vi "NI VeriStand - Get System Node Children.vi"(8 "error in (no error)":errorcluster, 10 "Node":string, 11 "WorkspaceManager in":T3) -> (0 "error out":errorcluster {"code" format="%.0x"}, 2 "Nodes":T1[](array[typedef]), 3 "WorkspaceManager out":T3)   [LabVIEW 2020, in "NI_VS Workspace ExecutionAPI.lvlib"]
doc: "Returns information about the nodes directly under the specified system node."
uses:
  <vilib>/NI VeriStand/Execution/Workspace/NI_VS Workspace ExecutionAPI.lvlib
  <vilib>/NI VeriStand/Execution/Workspace/WorkspaceAPI.ctl
  NationalInstruments.VeriStand.ClientAPI
  <vilib>/NI VeriStand/Execution/Workspace/NodeInfo.ctl
  <vilib>/NI VeriStand/Execution/Workspace/Waveform Data Type.ctl
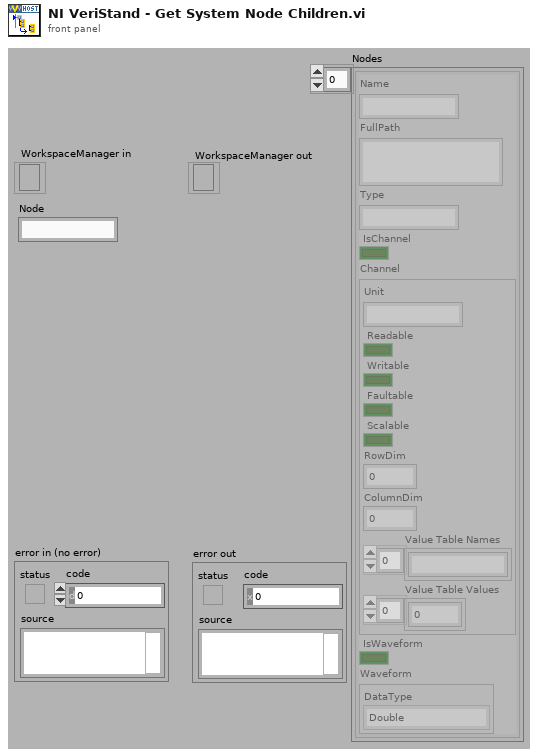
[diagram p1: front panel]
types:
  T1 = typedef "NI_VS Workspace ExecutionAPI.lvlib/NodeInfo.ctl" = cluster{"Name":string, "FullPath":string, "Type":string, "IsChannel":bool, "Channel":cluster{"Unit":string, "Readable":bool, "Writable":bool, "Faultable":bool, "Scalable":bool, "RowDim":u32, "ColumnDim":u32, "Value Table Names":string[], "Value Table Values":dbl[]}, "IsWaveform":bool, "Waveform":cluster{"DataType":T2}}
  T2 = typedef "NI_VS Workspace ExecutionAPI.lvlib/Waveform Data Type.ctl" = enum16{"Double", "ComplexDouble"}
  T3 = typedef "NI_VS Workspace ExecutionAPI.lvlib/WorkspaceAPI.ctl" = refnum<k24>
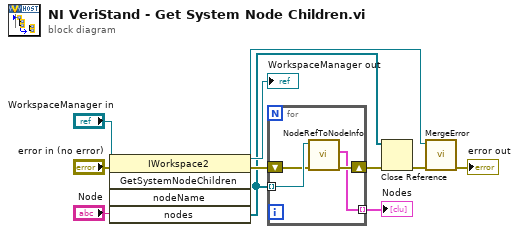
[diagram p0: block diagram]
diagram:
  n1 = invoke class="IWorkspace2" method="GetSystemNodeChildren"(reference="WorkspaceManager in", error in="error in (no error)", "nodeName"="Node") -> (reference out=→"WorkspaceManager out":T3, error out=w5:errorcluster, "GetSystemNodeChildren"=w4:refnum<k24>, "nodes"=w2:refnum<k24>[])  [unwired: 2 in, 1 out]
  n2 = for {
    tunnel: w2 -> [w15] mode=indexing
    shift-right: [w13] -> w7
    shift-left: w5 -> [w14]
    tunnel: [w12] -> w3 mode=indexing
    n3 = call <vilib>:"NodeRefToNodeInfo.vi"("error in (no error)"=w14, "Node"=w15) -> ("error out"=w13:errorcluster, "NodeInfo"=w12:T1)  [unwired: 8 out]
  }
  "Nodes" <- w3
  n4 = Close Reference(reference=w2, error in (no error)=w7) -> (error out=w6:errorcluster)
  n5 = call <vilib>:"MergeError.vi"("error in (no error)"=w6, "Error"=w4) -> ("error out"=→"error out":errorcluster)  [unwired: 9 out]
